vi "Get Named Ranges.vi"(8 "error in":errorcluster, 10 "Sheet Name":string, 11 "SpreadsheetDoc in":refnum<k24>) -> (0 "error out":errorcluster, 1 "Cells":cluster{"Cells":variant[][]}[](array[cluster]), 2 "Range Names":string[](array[string]), 3 "SpreadsheetDoc out":refnum<k24>)   [LabVIEW 2019, in "Open Xml.lvlib"]
uses:
  Open Xml.lvlib
  D:/git/Open-Xml-LabVIEW/Source/DocumentFormat.OpenXml.dll
  DocumentFormat.OpenXml.dll
  D:/git/Open-Xml-LabVIEW/Source/DocumentFormat.OpenXml.Framework.dll
  DocumentFormat.OpenXml.Framework.dll
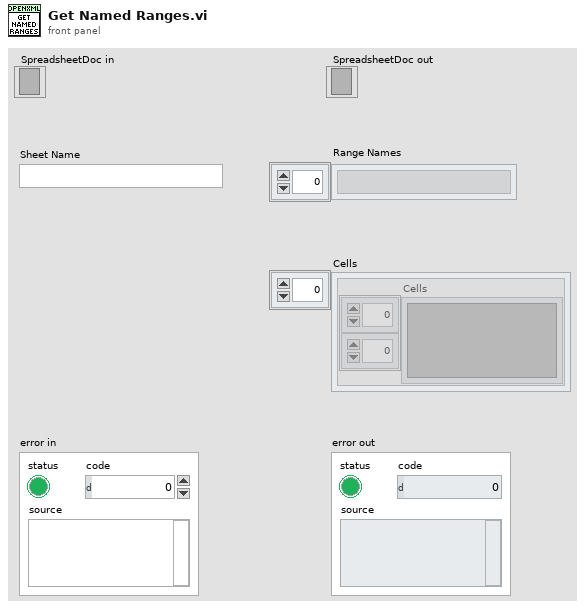
[diagram p1: front panel]
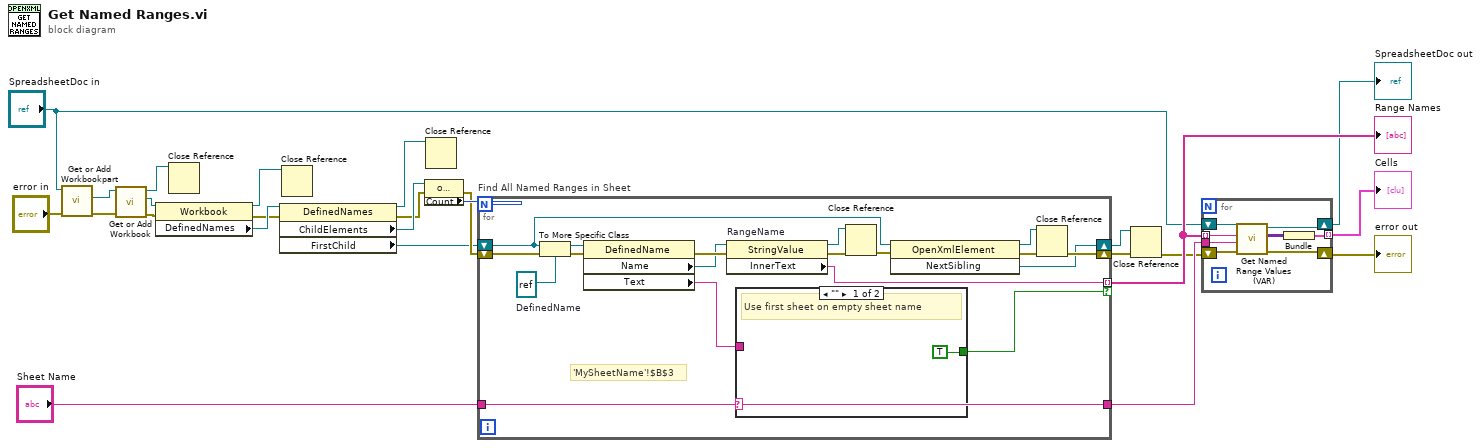
[diagram p0: block diagram]
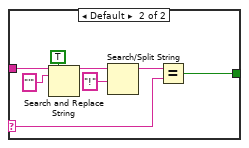
[diagram p2: hidden frame]
diagram:
  n1 = call "Get or Add Workbookpart.vi"("error in"="error in", "SpreadsheetDoc in"="SpreadsheetDoc in") -> ("error out"=w12:errorcluster, "WorkbookPart"=w9:refnum<k24>)  [unwired: 7 in, 1 out]
  n2 = call "Get or Add Workbook.vi"("error in"=w12, "Workbookpart in"=w9) -> ("error out"=w13:errorcluster, "Workbook"=w10:refnum<k24>, "Workbookpart out"=w2:refnum<k24>)  [unwired: 7 in]
  n3 = property class="Workbook"(reference=w10, error in=w13) -> (reference out=w24:refnum<k24>, error out=w11:errorcluster, "DefinedNames"=w25:refnum<k24>)
  n4 = Close Reference(reference=w2) -> ()  [unwired: 1 in, 1 out]
  n5 = property class="DefinedNames"(reference=w25, error in=w11) -> (reference out=w23:refnum<k24>, error out=w6:errorcluster, "ChildElements"=w8:refnum<k24>, "FirstChild"=w3:refnum<k24>)
  n6 = Close Reference(reference=w24) -> ()  [unwired: 1 in, 1 out]
  n7 = property class="OpenXmlElementList"(reference=w8, error in=w6) -> (error out=w5:errorcluster, "Count"=w7:i32)  [unwired: 1 out]
  n8 = Close Reference(reference=w23) -> ()  [unwired: 1 in, 1 out]
  n9 = for "Find All Named Ranges in Sheet" {
    N: w7 -> [_]
    shift-right: [w41] -> w20
    shift-left: w5 -> [w32]
    tunnel: "Sheet Name" -> [w33]
    shift-right: [w39] -> w16
    shift-left: w3 -> [w26]
    tunnel: [w35] -> w21 mode=indexing if=w34
    tunnel: [w33] -> w18
    w40 = refnum<k24> refnum  # DefinedName
    # "'MySheetName'!$B$3"
    n10 = To More Specific Class(target class=w40, reference=w26, error in=w32) -> (specific class reference=w43:refnum<k24>, error out=w42:errorcluster)
    n11 = property class="DefinedName"(reference=w43, error in=w42) -> (error out=w31:errorcluster, "Name"=w29:refnum<k24>, "Text"=w30:string)  [unwired: 1 out]
    n12 = property on="RangeName" class="StringValue"(reference=w29, error in=w31) -> (reference out=w38:refnum<k24>, error out=w28:errorcluster, "InnerText"=w35:string)
    n13 = case shown="\"\"" w33 {
      selector: w33 -> [_ w47]
      tunnel: [TRUE w48] -> w34
      tunnel: w30 -> [_ w45]
      frame "" {
        # "Use first sheet on empty sheet name"
      }
      frame Default {
        n14 = Search and Replace String(replace all?=TRUE ("replace all? (F)"), input string=w45, search string="'") -> (result string=w52:string)  [unwired: 5 in, 3 out]
        n15 = Search/Split String(string=w52, search string/char (-)="!") -> (substring before match=w46:string)  [unwired: 1 in, 2 out]
        n16 = Equal?(x=w46, y=w47) -> (x = y?=w48:bool)
      }
    }
    n17 = Close Reference(reference=w38, error in (no error)=w28) -> (error out=w27:errorcluster)
    n18 = invoke class="OpenXmlElement" method="NextSibling"(reference=w26, error in=w27) -> (reference out=w36:refnum<k24>, error out=w37:errorcluster, "NextSibling"=w39:refnum<k24>)  [unwired: 1 in]
    n19 = Close Reference(reference=w36, error in (no error)=w37) -> (error out=w41:errorcluster)
  }
  "Range Names" <- w21
  n20 = Close Reference(reference=w16, error in (no error)=w20) -> (error out=w17:errorcluster)
  n21 = for {
    tunnel: w21 -> [w60] mode=indexing
    shift-right: [w57] -> w19
    shift-left: w17 -> [w59]
    tunnel: w18 -> [w58]
    shift-right: [w54] -> w4
    shift-left: "SpreadsheetDoc in" -> [w53]
    tunnel: [w55] -> w15 mode=indexing
    n22 = call "Get Named Range Values (VAR).vi"("error in"=w59, "Sheet Name"=w58, "Named Range Identifier"=w60, "SpreadsheetDoc in"=w53) -> ("error out"=w57:errorcluster, "Cells"=w56:variant[][], "SpreadsheetDoc out"=w54:refnum<k24>)  [unwired: 5 in]
    n23 = Bundle("Cells"=w56) -> (w55:cluster{"Cells":variant[][]})  [unwired: 1 in]
  }
  "SpreadsheetDoc out" <- w4
  "error out" <- w19
  "Cells" <- w15
